vi "CarWashControllerClient.vi"() -> ()   [LabVIEW 2021]
uses:
  CarWashControllerStates.ctl
  <vilib>/regexp/Match Regular Expression.xnode
panel:
  out "error out":errorcluster
  in  "btnStop":bool
  out "tblink 4":bool
  out "tblink 3":bool
  out "tblink 2":bool
  out "tblink1":bool
  out "Seconds":string
  out "Minute":string
  out "Hour":string
  out "AM/PM":string
  out "Date":string
  out "Time":dbl
  out "Remaining Time":dbl
  in  "btnEconomy":bool
  in  "btnDeluxe":bool
  out "carState":string
  in  "LED-VOP":bool
  in  "LED-AD":bool
  in  "LED-CWR":bool
  in  "LED-MHPW":bool
  in  "LED-UBW":bool
  in  "LED-SA":bool
  out "CarWash Details":string
  out "CarWash Bytes":string
  out "Elapsed time":dbl
  in  "Set time":dbl
  in  "Air Dry Position Switch":bool
  in  "Main Wash Position Switch":bool
  in  "Under Body Wash Position \nSwitch":bool
  # "Purchase Selection"
  # "Select Your Wash"
  # "Remaining Time"
  # "Car Wash simulation switch"
  # "Air Dry\nPosition\nSwitch"
  # "Main Wash\nPosition \nSwitch"
  # "Deluxe Wash"
  # "Economy Wash"
  # "Car Wash Indicators"
  # "Under Body Wash"
  # "Soap Application"
  # "Main High Pressure Wash"
  # "Clear Water Rinse"
  # "Air Dry"
  # "Vehicle Out of Position"
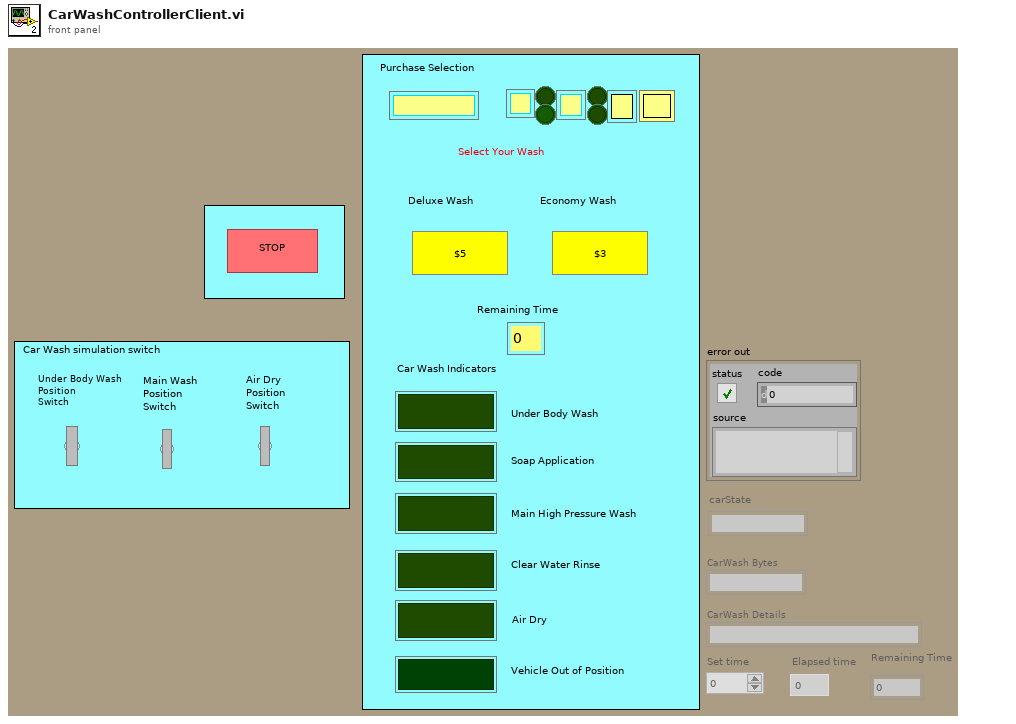
[diagram p1: front panel]
types:
  T1 = typedef "CarWashControllerStates.ctl" = enum16{"Start", "CarWashSelection", "Underbody Wash", "Soap Application", "Main High-Pressure Wash", "Clear Water rinse", "Air Dry Cycle", "Format", "Transmission", "End"}
  T2 = enum8{"Enabled", "Disabled", "Disabled and Grayed Out"}
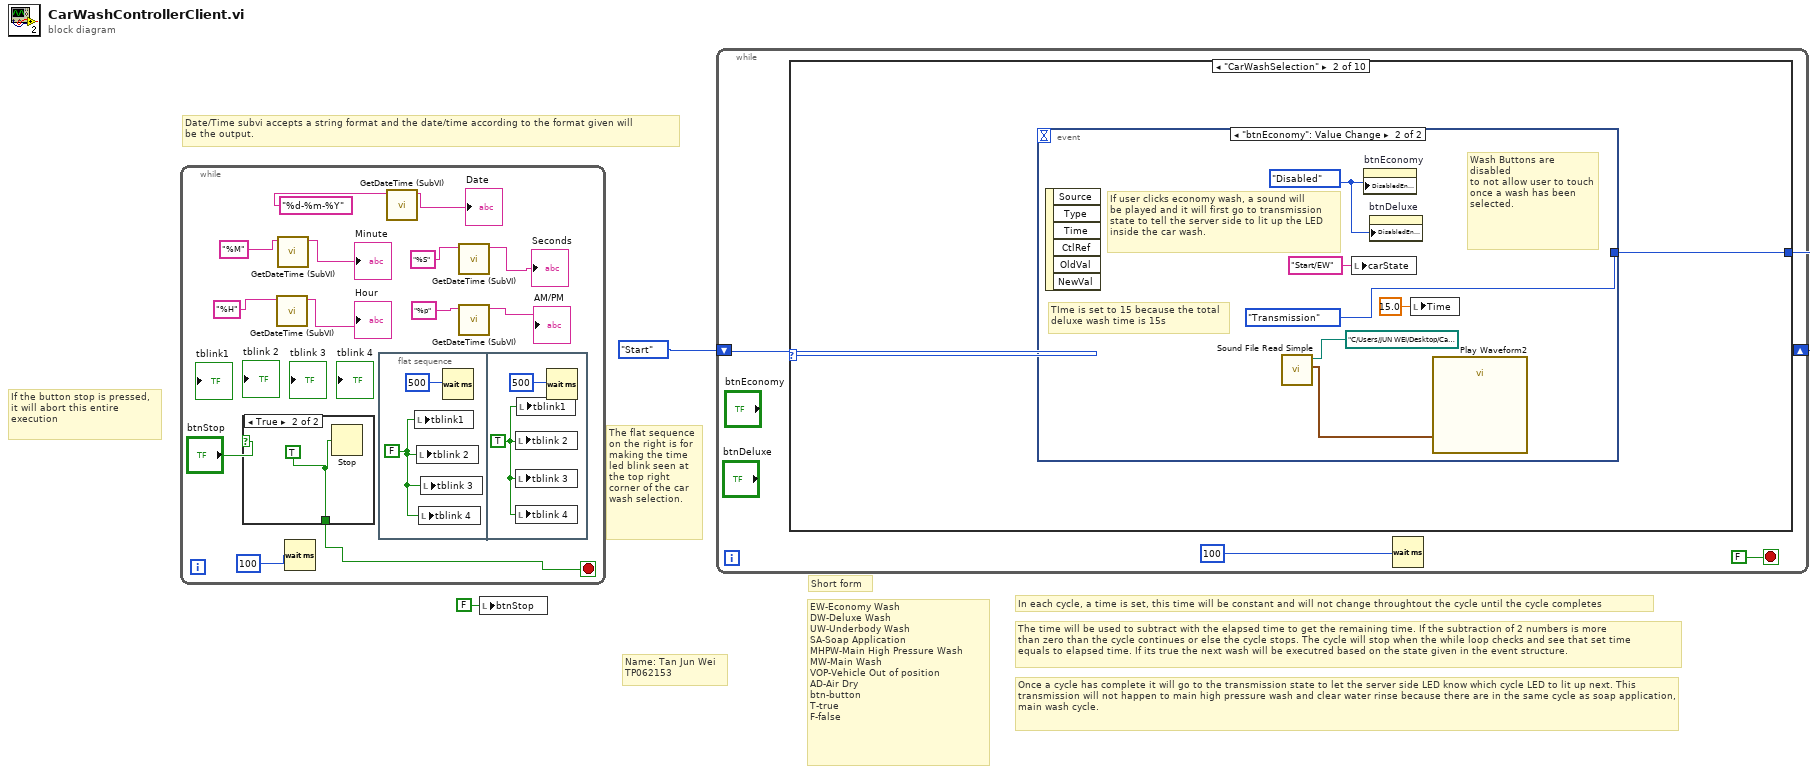
[diagram p0: block diagram]
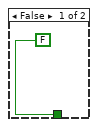
[diagram p2: hidden frame]
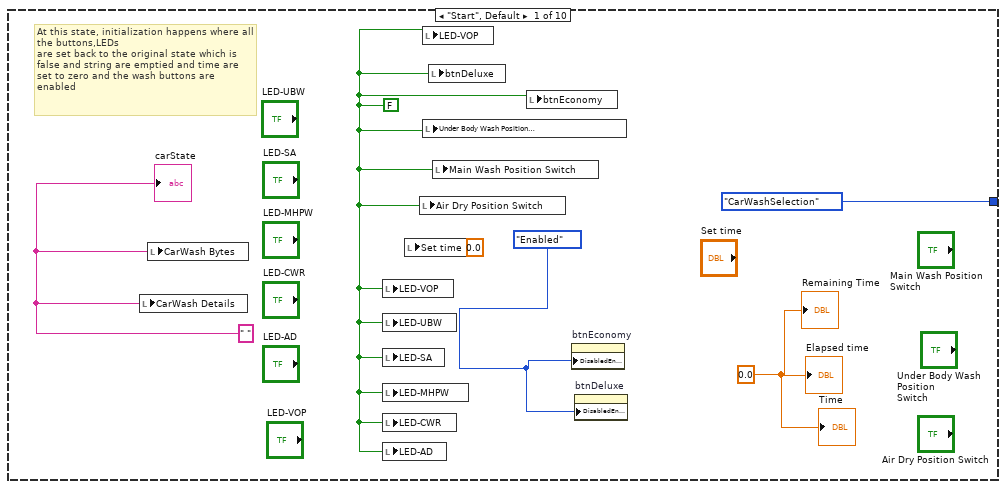
[diagram p3: hidden frame]
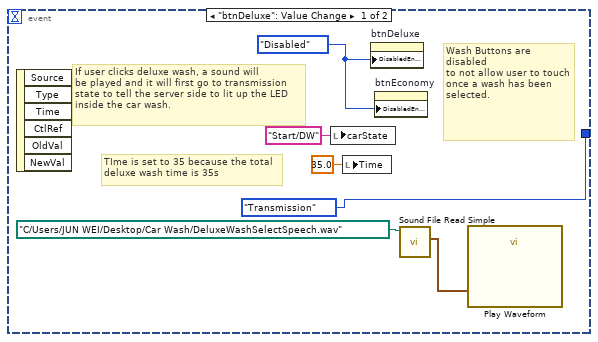
[diagram p4: hidden frame]
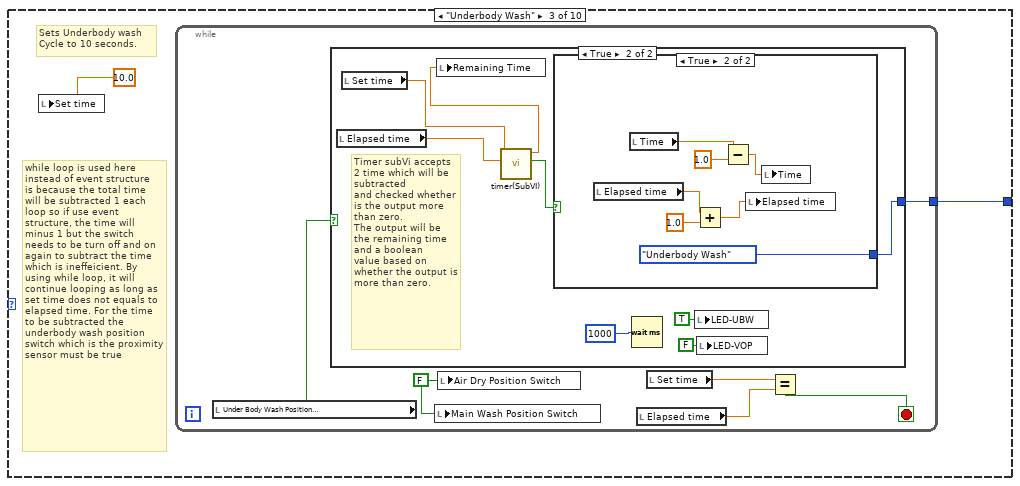
[diagram p5: hidden frame]
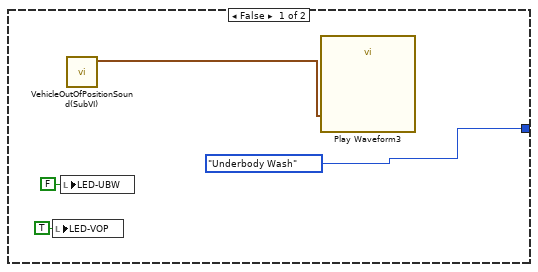
[diagram p6: hidden frame]
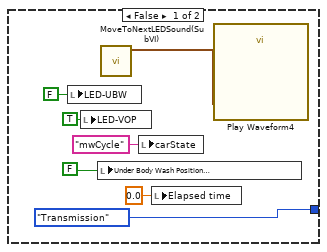
[diagram p7: hidden frame]
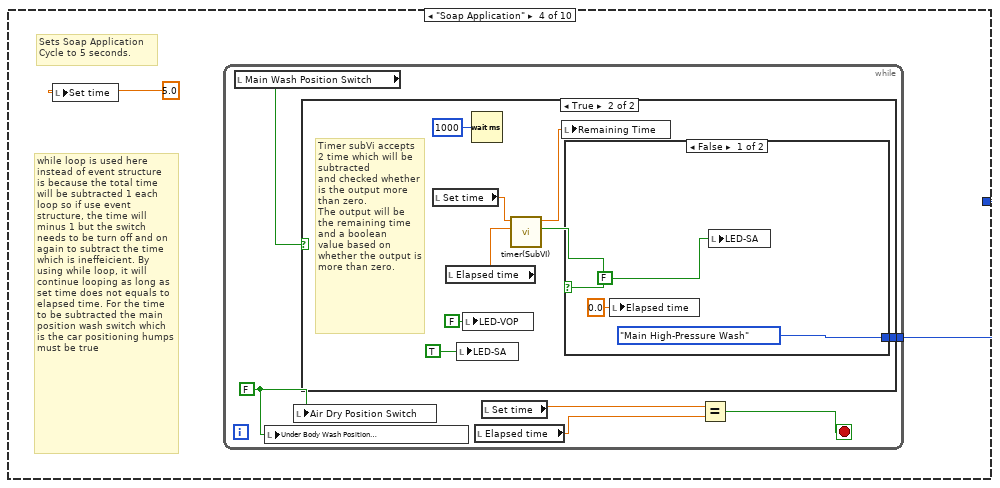
[diagram p8: hidden frame]
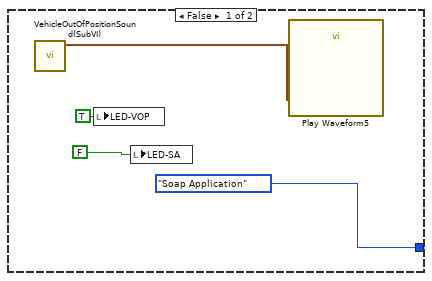
[diagram p9: hidden frame]
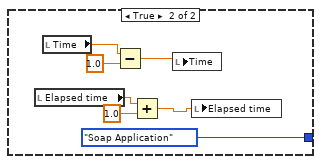
[diagram p10: hidden frame]
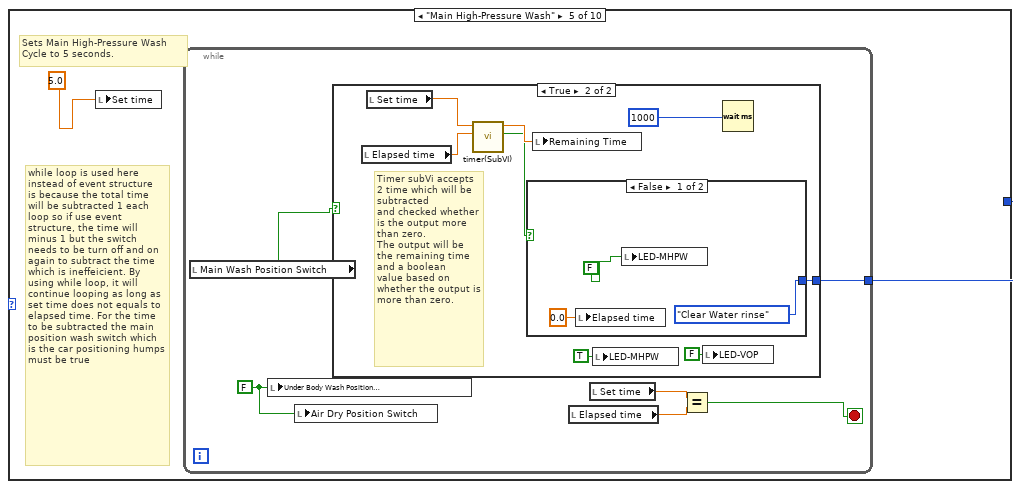
[diagram p11: hidden frame]
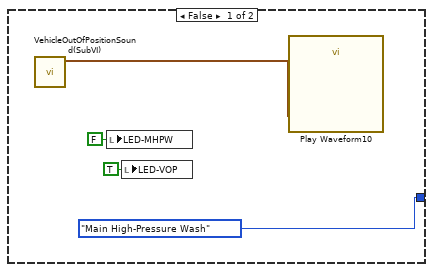
[diagram p12: hidden frame]
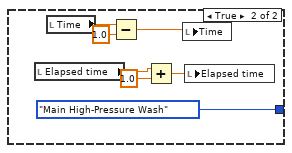
[diagram p13: hidden frame]
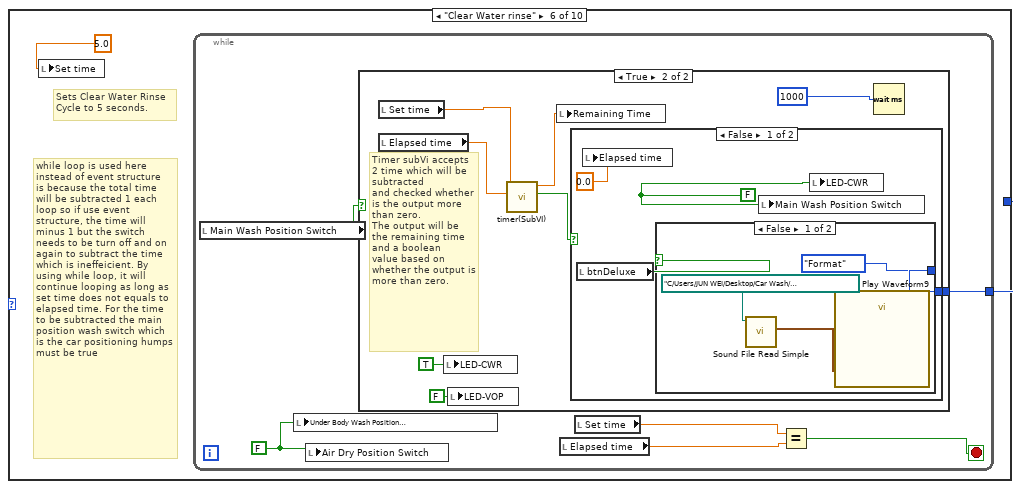
[diagram p14: hidden frame]
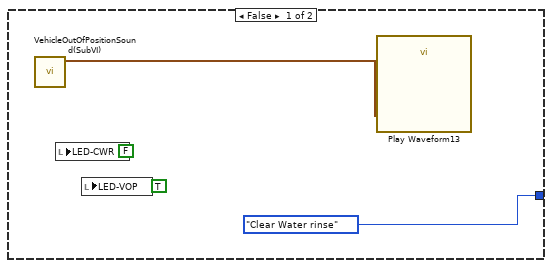
[diagram p15: hidden frame]
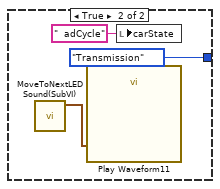
[diagram p16: hidden frame]
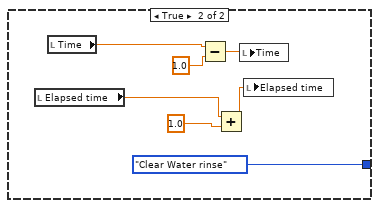
[diagram p17: hidden frame]
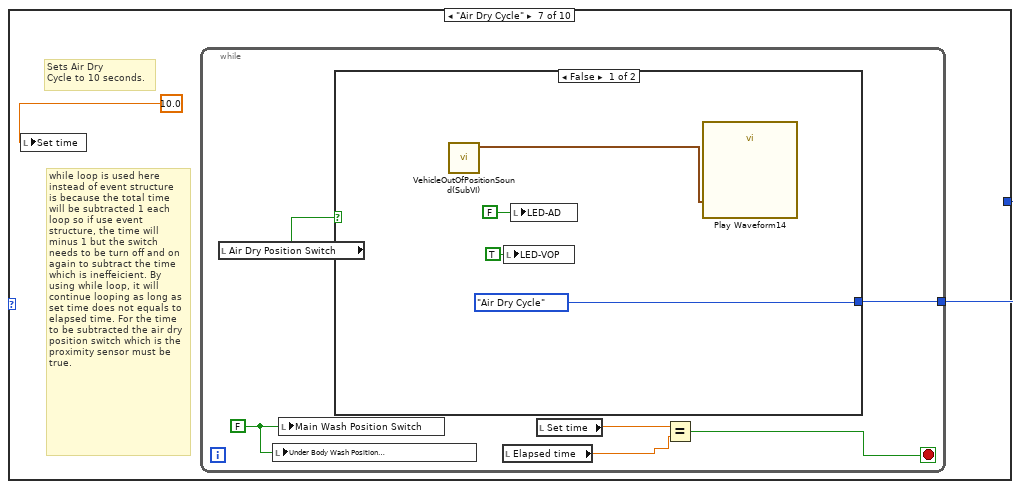
[diagram p18: hidden frame]
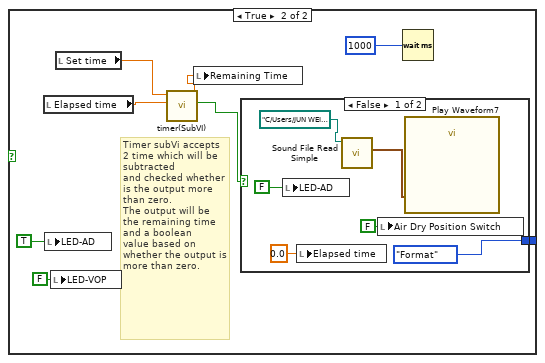
[diagram p19: hidden frame]
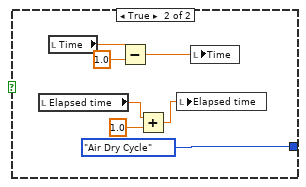
[diagram p20: hidden frame]
diagram:
  # "Short form"
  # "EW-Economy Wash\nDW-Deluxe Wash\nUW-Underbody Wash\nSA-Soap Application\nMHPW-Main High Pressure Wash\nMW-Main Wash\nVOP-Vehicle Out of position\nAD-Air Dry\nbtn-button\nT-true\nF-false"
  # "Name: Tan Jun Wei\nTP062153"
  # "Date/Time subvi accepts a string format and the date/time according to the format given will \nbe the output."
  # "The flat sequence on the right is for making the time led blink seen at the top right corner of the car wash selection."
  # "If the button stop is pressed, it will abort this entire execution"
  # "Once a cycle has complete it will go to the transmission state to let the server side LED know which cycle LED to lit up next. This transmission will not happen to main high pressure wash and clear water rinse because there are in the same cycle as soap application, main wash cycle."
  # "The time will be used to subtract with the elapsed time to get the remaining time. If the subtraction of 2 numbers is more \nthan zero than the cycle continues or else the cycle stops. The cycle will stop when the while loop checks and see that set time\nequals to elapsed time. If its true the next wash will be executred based on the state given in the event structure."
  # "In each cycle, a time is set, this time will be constant and will not change throughtout the cycle until the cycle completes"
  n1 = while {
    stop <- w3 stop-if-true
    n2 = case shown="True" "btnStop" {
      tunnel: [FALSE w17] -> w3
      frame False {
      }
      frame True {
        w17 = TRUE
        n3 = Stop(stop? (T)=w17) -> ()
      }
    }
    n4 = call "GetDateTime (SubVI).vi"("time format string (%c)"="%H") -> ("date/time string"=→"Hour":string)  [unwired: 10 in]
    n5 = call "GetDateTime (SubVI).vi"("time format string (%c)"="%M") -> ("date/time string"=→"Minute":string)  [unwired: 10 in]
    n6 = Wait (ms)(milliseconds to wait=u32 100 ("millisecond timer value")) -> ()  [unwired: 1 out]
    n7 = flat-sequence {
      frame #0 {
        w19 = FALSE ("blink 2")
        n8 = local write "tblink1"(w19) -> ()
        n9 = local write "tblink 2"(w19) -> ()
        n10 = local write "tblink 4"(w19) -> ()
        n11 = local write "tblink 3"(w19) -> ()
        n12 = Wait (ms)(milliseconds to wait=u32 500 ("millisecond timer value")) -> ()  [unwired: 1 out]
      }
      frame #1 {
        w21 = TRUE ("blink 2")
        n13 = local write "tblink 2"(w21) -> ()
        n14 = local write "tblink 3"(w21) -> ()
        n15 = local write "tblink 4"(w21) -> ()
        n16 = local write "tblink1"(w21) -> ()
        n17 = Wait (ms)(milliseconds to wait=u32 500 ("millisecond timer value")) -> ()  [unwired: 1 out]
      }
    }
    n18 = call "GetDateTime (SubVI).vi"("time format string (%c)"="%d-%m-%Y") -> ("date/time string"=→"Date":string)  [unwired: 10 in]
    n19 = call "GetDateTime (SubVI).vi"("time format string (%c)"="%S") -> ("date/time string"=→"Seconds":string)  [unwired: 10 in]
    n20 = call "GetDateTime (SubVI).vi"("time format string (%c)"="%p") -> ("date/time string"=→"AM/PM":string)  [unwired: 10 in]
  }
  n21 = local write "btnStop"(FALSE ("btnStop")) -> ()
  n22 = while {
    shift-right: [w23] -> _
    shift-left: CarWashControllerStates."Start" -> [w25]
    stop <- FALSE stop-if-true
    n23 = case shown="\"CarWashSelection\"" w25 {
      tunnel: [CarWashControllerStates."CarWashSelection" w32 w46 w79 w109 w139 w176 CarWashControllerStates."Transmission" w230 CarWashControllerStates."Start"] -> w23
      frame "Start", Default {
        w27 = 0.0 ("Remaining Time")
        w28 = " " ("carState")
        w29 = T2."Enabled" ("Disabled")
        w26 = FALSE ("btnEconomy")
        # "At this state, initialization happens where all the buttons,LEDs\nare set back to the original state which is false and string are emptied and time are set to zero and the wash buttons are enabled"
        n24 = local write "CarWash Details"(w28) -> ()
        n25 = local write "CarWash Bytes"(w28) -> ()
        n26 = local write "LED-VOP"(w26) -> ()
        n27 = local write "LED-UBW"(w26) -> ()
        n28 = local write "LED-SA"(w26) -> ()
        n29 = local write "LED-MHPW"(w26) -> ()
        n30 = local write "LED-CWR"(w26) -> ()
        n31 = local write "LED-AD"(w26) -> ()
        n32 = local write "Set time"(0.0 ("Set time")) -> ()
        n33 = local write "Air Dry Position Switch"(w26) -> ()
        n34 = local write "LED-VOP"(w26) -> ()
        n35 = local write "Under Body Wash Position \nSwitch"(w26) -> ()
        n36 = local write "btnDeluxe"(w26) -> ()
        n37 = local write "Main Wash Position Switch"(w26) -> ()
        n38 = local write "btnEconomy"(w26) -> ()
        n39 = property on="btnEconomy" class="Bool (strict)"("DisabledEnum"=w29) -> ()  [unwired: 2 in, 2 out]
        n40 = property on="btnDeluxe" class="Bool (strict)"("DisabledEnum"=w29) -> ()  [unwired: 2 in, 2 out]
        "carState" <- w28
        "Remaining Time" <- w27
        "Elapsed time" <- w27
        "Time" <- w27
      }
      frame "CarWashSelection" {
        n41 = event shown="[1] \"btnEconomy\": Value Change" {
          selector: _ -> [_ _]
          dyn-events: _ -> [_ _]
          timeout: _ -> [_ _]
          tunnel: [CarWashControllerStates."Transmission" CarWashControllerStates."Transmission"] -> w32
          event "btnDeluxe": Value Change {
            w35 = T2."Disabled" ("Disabled")
            # "TIme is set to 35 because the total\ndeluxe wash time is 35s"
            # "Wash Buttons are disabled\nto not allow user to touch once a wash has been selected."
            # "If user clicks deluxe wash, a sound will\nbe played and it will first go to transmission\nstate to tell the server side to lit up the LED \ninside the car wash."
            n42 = event-data() -> ()  [unwired: 1 in, 6 out]
            n43 = local write "carState"("Start/DW" ("carState")) -> ()
            n44 = local write "Time"(35.0 ("Time")) -> ()
            n45 = property on="btnDeluxe" class="Bool (strict)"("DisabledEnum"=w35) -> ()  [unwired: 2 in, 2 out]
            n46 = property on="btnEconomy" class="Bool (strict)"("DisabledEnum"=w35) -> ()  [unwired: 2 in, 2 out]
            n47 = call <vilib>:"Sound File Read Simple.vi"("path"=path "C:/Users/JUN WEI/Desktop/Car Wash/DeluxeWashSelectSpeech.wav") -> ("data"=w33:waveform(dbl)[])  [unwired: 7 in, 3 out]
            n48 = call "Play Waveform"("Data"=w33) -> ()  [unwired: 18 in, 1 out]
          }
          event "btnEconomy": Value Change {
            w41 = T2."Disabled" ("Disabled")
            # "TIme is set to 15 because the total\ndeluxe wash time is 15s"
            # "Wash Buttons are disabled\nto not allow user to touch once a wash has been selected."
            # "If user clicks economy wash, a sound will\nbe played and it will first go to transmission\nstate to tell the server side to lit up the LED \ninside the car wash."
            n49 = event-data() -> ()  [unwired: 1 in, 6 out]
            n50 = call <vilib>:"Sound File Read Simple.vi"("path"=path "C:/Users/JUN WEI/Desktop/Car Wash/EconomyWashSelectSpeech.wav") -> ("data"=w40:waveform(dbl)[])  [unwired: 7 in, 3 out]
            n51 = local write "carState"("Start/EW" ("carState")) -> ()
            n52 = property on="btnEconomy" class="Bool (strict)"("DisabledEnum"=w41) -> ()  [unwired: 2 in, 2 out]
            n53 = property on="btnDeluxe" class="Bool (strict)"("DisabledEnum"=w41) -> ()  [unwired: 2 in, 2 out]
            n54 = local write "Time"(15.0 ("Time")) -> ()
            n55 = call "Play Waveform2"("Data"=w40) -> ()  [unwired: 18 in, 1 out]
          }
        }
      }
      frame "Underbody Wash" {
        # "Sets Underbody wash \nCycle to 10 seconds."
        # "while loop is used here\ninstead of event structure\nis because the total time will be subtracted 1 each loop so if use event structure, the time will  minus 1 but the switch needs to be turn off and on again to subtract the time which is ineffeicient. By using while loop, it will continue looping as long as set time does not equals to elapsed time. For the time to be subtracted the underbody wash position switch which is the proximity sensor must be true"
        n56 = local write "Set time"(10.0 ("Set time")) -> ()
        n57 = while {
          tunnel: [w51] -> w46
          stop <- w48 stop-if-true
          w47 = FALSE ("Air Dry Position Switch")
          n58 = local read "Under Body Wash Position \nSwitch"() -> (w52:bool)
          n59 = case shown="True" w52 {
            tunnel: [CarWashControllerStates."Underbody Wash" w57] -> w51
            frame False {
              n60 = local write "LED-VOP"(TRUE ("swVOP")) -> ()
              n61 = local write "LED-UBW"(FALSE ("Boolean")) -> ()
              n62 = call "VehicleOutOfPositionSound(SubVI).vi"() -> ("data"=w53:waveform(dbl)[])  [unwired: 11 in]
              n63 = call "Play Waveform3"("Data"=w53) -> ()  [unwired: 18 in, 1 out]
            }
            frame True {
              # "Timer subVi accepts\n2 time which will be subtracted\nand checked whether is the output more than zero.\nThe output will be the remaining time and a boolean \nvalue based on whether the output is more than zero."
              n64 = local read "Elapsed time"() -> (w63:dbl)
              n65 = local read "Set time"() -> (w64:dbl)
              n66 = call "timer(SubVI).vi"("Elapsed time"=w63, "Set time"=w64) -> ("Boolean"=w61:bool, "Remaining Time"=w62:dbl)  [unwired: 8 in]
              n67 = local write "Remaining Time"(w62) -> ()
              n68 = case shown="True" w61 {
                tunnel: [CarWashControllerStates."Transmission" CarWashControllerStates."Underbody Wash"] -> w57
                frame False {
                  n69 = local write "LED-UBW"(FALSE ("LED-UBW")) -> ()
                  n70 = local write "LED-VOP"(TRUE ("swVOP")) -> ()
                  n71 = local write "Under Body Wash Position \nSwitch"(FALSE ("s1")) -> ()
                  n72 = call "MoveToNextLEDSound(SubVI).vi"() -> ("data"=w65:waveform(dbl)[])  [unwired: 11 in]
                  n73 = local write "carState"("mwCycle" ("carState")) -> ()
                  n74 = local write "Elapsed time"(0.0 ("Elapsed time")) -> ()
                  n75 = call "Play Waveform4"("Data"=w65) -> ()  [unwired: 18 in, 1 out]
                }
                frame True {
                  n76 = local read "Elapsed time"() -> (w77:dbl)
                  n77 = local read "Time"() -> (w73:dbl)
                  n78 = Add(x=w77, y=1.0) -> (x+y=w76:dbl)
                  n79 = Subtract(x=w73, y=1.0) -> (x-y=w74:dbl)
                  n80 = local write "Elapsed time"(w76) -> ()
                  n81 = local write "Time"(w74) -> ()
                }
              }
              n82 = Wait (ms)(milliseconds to wait=u32 1000 ("millisecond timer value")) -> ()  [unwired: 1 out]
              n83 = local write "LED-UBW"(TRUE ("Boolean")) -> ()
              n84 = local write "LED-VOP"(FALSE ("swVOP")) -> ()
            }
          }
          n85 = local write "Main Wash Position Switch"(w47) -> ()
          n86 = local write "Air Dry Position Switch"(w47) -> ()
          n87 = local read "Elapsed time"() -> (w49:dbl)
          n88 = local read "Set time"() -> (w50:dbl)
          n89 = Equal?(x=w50, y=w49) -> (x = y?=w48:bool)
        }
      }
      frame "Soap Application" {
        # "Sets Soap Application \nCycle to 5 seconds."
        # "while loop is used here\ninstead of event structure\nis because the total time will be subtracted 1 each loop so if use event structure, the time will  minus 1 but the switch needs to be turn off and on again to subtract the time which is ineffeicient. By using while loop, it will continue looping as long as set time does not equals to elapsed time. For the time to be subtracted the main position wash switch which is the car positioning humps must be true"
        n90 = local write "Set time"(5.0 ("Set time")) -> ()
        n91 = while {
          tunnel: [w85] -> w79
          stop <- w82 stop-if-true
          w81 = FALSE ("Air Dry Position Switch")
          n92 = local read "Main Wash Position Switch"() -> (w86:bool)
          n93 = local write "Under Body Wash Position \nSwitch"(w81) -> ()
          n94 = local write "Air Dry Position Switch"(w81) -> ()
          n95 = case shown="True" w86 {
            tunnel: [CarWashControllerStates."Soap Application" w98] -> w85
            frame False {
              n96 = call "VehicleOutOfPositionSound(SubVI).vi"() -> ("data"=w87:waveform(dbl)[])  [unwired: 11 in]
              n97 = local write "LED-VOP"(TRUE ("swVOP")) -> ()
              n98 = local write "LED-SA"(FALSE ("Boolean")) -> ()
              n99 = call "Play Waveform5"("Data"=w87) -> ()  [unwired: 18 in, 1 out]
            }
            frame True {
              # "Timer subVi accepts\n2 time which will be subtracted\nand checked whether is the output more than zero.\nThe output will be the remaining time and a boolean \nvalue based on whether the output is more than zero."
              n100 = local read "Set time"() -> (w93:dbl)
              n101 = local read "Elapsed time"() -> (w94:dbl)
              n102 = local write "LED-SA"(TRUE ("Boolean 2")) -> ()
              n103 = local write "LED-VOP"(FALSE ("swVOP")) -> ()
              n104 = Wait (ms)(milliseconds to wait=u32 1000) -> ()  [unwired: 1 out]
              n105 = call "timer(SubVI).vi"("Elapsed time"=w94, "Set time"=w93) -> ("Boolean"=w91:bool, "Remaining Time"=w92:dbl)  [unwired: 8 in]
              n106 = local write "Remaining Time"(w92) -> ()
              n107 = case shown="False" w91 {
                tunnel: [CarWashControllerStates."Main High-Pressure Wash" CarWashControllerStates."Soap Application"] -> w98
                frame False {
                  n108 = local write "Elapsed time"(0.0 ("Elapsed time")) -> ()
                  n109 = local write "LED-SA"(FALSE ("s2")) -> ()
                }
                frame True {
                  n110 = local read "Elapsed time"() -> (w108:dbl)
                  n111 = local read "Time"() -> (w104:dbl)
                  n112 = Subtract(x=w104, y=1.0) -> (x-y=w102:dbl)
                  n113 = Add(x=w108, y=1.0) -> (x+y=w106:dbl)
                  n114 = local write "Time"(w102) -> ()
                  n115 = local write "Elapsed time"(w106) -> ()
                }
              }
            }
          }
          n116 = local read "Elapsed time"() -> (w83:dbl)
          n117 = local read "Set time"() -> (w84:dbl)
          n118 = Equal?(x=w84, y=w83) -> (x = y?=w82:bool)
        }
      }
      frame "Main High-Pressure Wash" {
        # "Sets Main High-Pressure Wash \nCycle to 5 seconds."
        # "while loop is used here\ninstead of event structure\nis because the total time will be subtracted 1 each loop so if use event structure, the time will  minus 1 but the switch needs to be turn off and on again to subtract the time which is ineffeicient. By using while loop, it will continue looping as long as set time does not equals to elapsed time. For the time to be subtracted the main position wash switch which is the car positioning humps must be true"
        n119 = local write "Set time"(5.0 ("Set time")) -> ()
        n120 = while {
          tunnel: [w113] -> w109
          stop <- w114 stop-if-true
          w111 = FALSE ("Under Body Wash Position \nSwitch")
          n121 = local read "Main Wash Position Switch"() -> (w112:bool)
          n122 = local write "Under Body Wash Position \nSwitch"(w111) -> ()
          n123 = local write "Air Dry Position Switch"(w111) -> ()
          n124 = case shown="True" w112 {
            tunnel: [CarWashControllerStates."Main High-Pressure Wash" w127] -> w113
            frame False {
              n125 = call "VehicleOutOfPositionSound(SubVI).vi"() -> ("data"=w117:waveform(dbl)[])  [unwired: 11 in]
              n126 = local write "LED-MHPW"(FALSE ("Boolean 3")) -> ()
              n127 = local write "LED-VOP"(TRUE ("swVOP")) -> ()
              n128 = call "Play Waveform10"("Data"=w117) -> ()  [unwired: 18 in, 1 out]
            }
            frame True {
              # "Timer subVi accepts\n2 time which will be subtracted\nand checked whether is the output more than zero.\nThe output will be the remaining time and a boolean \nvalue based on whether the output is more than zero."
              n129 = local read "Elapsed time"() -> (w124:dbl)
              n130 = local read "Set time"() -> (w123:dbl)
              n131 = call "timer(SubVI).vi"("Elapsed time"=w124, "Set time"=w123) -> ("Boolean"=w121:bool, "Remaining Time"=w122:dbl)  [unwired: 8 in]
              n132 = case shown="False" w121 {
                tunnel: [CarWashControllerStates."Clear Water rinse" CarWashControllerStates."Main High-Pressure Wash"] -> w127
                frame False {
                  n133 = local write "Elapsed time"(0.0 ("Elapsed time")) -> ()
                  n134 = local write "LED-MHPW"(FALSE ("s2")) -> ()
                }
                frame True {
                  n135 = local read "Elapsed time"() -> (w137:dbl)
                  n136 = local read "Time"() -> (w135:dbl)
                  n137 = Subtract(x=w135, y=1.0) -> (x-y=w132:dbl)
                  n138 = Add(x=w137, y=1.0) -> (x+y=w133:dbl)
                  n139 = local write "Time"(w132) -> ()
                  n140 = local write "Elapsed time"(w133) -> ()
                }
              }
              n141 = local write "Remaining Time"(w122) -> ()
              n142 = local write "LED-MHPW"(TRUE ("Boolean 3")) -> ()
              n143 = local write "LED-VOP"(FALSE ("swVOP")) -> ()
              n144 = Wait (ms)(milliseconds to wait=u32 1000 ("millisecond timer value")) -> ()  [unwired: 1 out]
            }
          }
          n145 = local read "Elapsed time"() -> (w115:dbl)
          n146 = local read "Set time"() -> (w116:dbl)
          n147 = Equal?(x=w116, y=w115) -> (x = y?=w114:bool)
        }
      }
      frame "Clear Water rinse" {
        # "while loop is used here\ninstead of event structure\nis because the total time will be subtracted 1 each loop so if use event structure, the time will  minus 1 but the switch needs to be turn off and on again to subtract the time which is ineffeicient. By using while loop, it will continue looping as long as set time does not equals to elapsed time. For the time to be subtracted the main position wash switch which is the car positioning humps must be true"
        # "Sets Clear Water Rinse \nCycle to 5 seconds."
        n148 = local write "Set time"(5.0 ("Set time")) -> ()
        n149 = while {
          tunnel: [w142] -> w139
          stop <- w144 stop-if-true
          w141 = FALSE ("Air Dry Position Switch")
          n150 = local read "Main Wash Position Switch"() -> (w143:bool)
          n151 = local write "Under Body Wash Position \nSwitch"(w141) -> ()
          n152 = local write "Air Dry Position Switch"(w141) -> ()
          n153 = case shown="True" w143 {
            tunnel: [CarWashControllerStates."Clear Water rinse" w156] -> w142
            frame False {
              n154 = call "VehicleOutOfPositionSound(SubVI).vi"() -> ("data"=w147:waveform(dbl)[])  [unwired: 11 in]
              n155 = local write "LED-CWR"(FALSE ("Boolean 4")) -> ()
              n156 = local write "LED-VOP"(TRUE ("swVOP")) -> ()
              n157 = call "Play Waveform13"("Data"=w147) -> ()  [unwired: 18 in, 1 out]
            }
            frame True {
              # "Timer subVi accepts\n2 time which will be subtracted\nand checked whether is the output more than zero.\nThe output will be the remaining time and a boolean \nvalue based on whether the output is more than zero."
              n158 = local read "Set time"() -> (w151:dbl)
              n159 = local read "Elapsed time"() -> (w152:dbl)
              n160 = local write "LED-CWR"(TRUE ("Boolean 4")) -> ()
              n161 = local write "LED-VOP"(FALSE ("swVOP")) -> ()
              n162 = call "timer(SubVI).vi"("Elapsed time"=w152, "Set time"=w151) -> ("Boolean"=w154:bool, "Remaining Time"=w153:dbl)  [unwired: 8 in]
              n163 = local write "Remaining Time"(w153) -> ()
              n164 = case shown="False" w154 {
                tunnel: [w162 CarWashControllerStates."Clear Water rinse"] -> w156
                frame False {
                  w161 = FALSE ("s2")
                  n165 = local read "btnDeluxe"() -> (w160:bool)
                  n166 = local write "Elapsed time"(0.0 ("Elapsed time")) -> ()
                  n167 = case shown="False" w160 {
                    tunnel: [CarWashControllerStates."Format" CarWashControllerStates."Transmission"] -> w162
                    frame False {
                      n168 = call <vilib>:"Sound File Read Simple.vi"("path"=path "C:/Users/JUN WEI/Desktop/Car Wash/EconomyWashExitSpeech.wav") -> ("data"=w164:waveform(dbl)[])  [unwired: 7 in, 3 out]
                      n169 = call "Play Waveform9"("Data"=w164) -> ()  [unwired: 18 in, 1 out]
                    }
                    frame True {
                      n170 = call "MoveToNextLEDSound(SubVI).vi"() -> ("data"=w166:waveform(dbl)[])  [unwired: 11 in]
                      n171 = call "Play Waveform11"("Data"=w166) -> ()  [unwired: 18 in, 1 out]
                      n172 = local write "carState"("  adCycle" ("carState")) -> ()
                    }
                  }
                  n173 = local write "Main Wash Position Switch"(w161) -> ()
                  n174 = local write "LED-CWR"(w161) -> ()
                }
                frame True {
                  n175 = local read "Elapsed time"() -> (w174:dbl)
                  n176 = local read "Time"() -> (w170:dbl)
                  n177 = Subtract(x=w170, y=1.0) -> (x-y=w171:dbl)
                  n178 = Add(x=w174, y=1.0) -> (x+y=w173:dbl)
                  n179 = local write "Time"(w171) -> ()
                  n180 = local write "Elapsed time"(w173) -> ()
                }
              }
              n181 = Wait (ms)(milliseconds to wait=u32 1000 ("millisecond timer value")) -> ()  [unwired: 1 out]
            }
          }
          n182 = local read "Elapsed time"() -> (w145:dbl)
          n183 = local read "Set time"() -> (w146:dbl)
          n184 = Equal?(x=w146, y=w145) -> (x = y?=w144:bool)
        }
      }
      frame "Air Dry Cycle" {
        # "Sets Air Dry  \nCycle to 10 seconds."
        # "while loop is used here\ninstead of event structure\nis because the total time will be subtracted 1 each loop so if use event structure, the time will  minus 1 but the switch needs to be turn off and on again to subtract the time which is ineffeicient. By using while loop, it will continue looping as long as set time does not equals to elapsed time. For the time to be subtracted the air dry position switch which is the proximity sensor must be true."
        n185 = local write "Set time"(10.0 ("Set time")) -> ()
        n186 = while {
          tunnel: [w182] -> w176
          stop <- w179 stop-if-true
          w178 = FALSE ("Main Wash Position Switch")
          n187 = local read "Air Dry Position Switch"() -> (w183:bool)
          n188 = local write "Under Body Wash Position \nSwitch"(w178) -> ()
          n189 = local write "Main Wash Position Switch"(w178) -> ()
          n190 = case shown="False" w183 {
            tunnel: [CarWashControllerStates."Air Dry Cycle" w194] -> w182
            frame False {
              n191 = call "VehicleOutOfPositionSound(SubVI).vi"() -> ("data"=w184:waveform(dbl)[])  [unwired: 11 in]
              n192 = local write "LED-VOP"(TRUE ("swVOP")) -> ()
              n193 = local write "LED-AD"(FALSE ("Boolean 5")) -> ()
              n194 = call "Play Waveform14"("Data"=w184) -> ()  [unwired: 18 in, 1 out]
            }
            frame True {
              # "Timer subVi accepts\n2 time which will be subtracted\nand checked whether is the output more than zero.\nThe output will be the remaining time and a boolean \nvalue based on whether the output is more than zero."
              n195 = local read "Elapsed time"() -> (w189:dbl)
              n196 = local write "LED-AD"(TRUE ("Boolean 5")) -> ()
              n197 = local write "LED-VOP"(FALSE ("swVOP")) -> ()
              n198 = local read "Set time"() -> (w188:dbl)
              n199 = call "timer(SubVI).vi"("Elapsed time"=w189, "Set time"=w188) -> ("Boolean"=w191:bool, "Remaining Time"=w190:dbl)  [unwired: 8 in]
              n200 = local write "Remaining Time"(w190) -> ()
              n201 = case shown="False" w191 {
                tunnel: [CarWashControllerStates."Format" CarWashControllerStates."Air Dry Cycle"] -> w194
                frame False {
                  n202 = local write "LED-AD"(FALSE ("Boolean 5")) -> ()
                  n203 = local write "Elapsed time"(0.0 ("Elapsed time")) -> ()
                  n204 = call <vilib>:"Sound File Read Simple.vi"("path"=path "C:/Users/JUN WEI/Desktop/Car Wash/DeluxeWashExitSpeech.wav") -> ("data"=w196:waveform(dbl)[])  [unwired: 7 in, 3 out]
                  n205 = local write "Air Dry Position Switch"(FALSE ("s3")) -> ()
                  n206 = call "Play Waveform7"("Data"=w196) -> ()  [unwired: 18 in, 1 out]
                }
                frame True {
                  n207 = local read "Elapsed time"() -> (w208:dbl)
                  n208 = local read "Time"() -> (w203:dbl)
                  n209 = Subtract(x=w203, y=1.0) -> (x-y=w202:dbl)
                  n210 = Add(x=w208, y=1.0) -> (x+y=w206:dbl)
                  n211 = local write "Elapsed time"(w206) -> ()
                  n212 = local write "Time"(w202) -> ()
                }
              }
              n213 = Wait (ms)(milliseconds to wait=u32 1000 ("millisecond timer value")) -> ()  [unwired: 1 out]
            }
          }
          n214 = local read "Elapsed time"() -> (w180:dbl)
          n215 = local read "Set time"() -> (w181:dbl)
          n216 = Equal?(x=w181, y=w180) -> (x = y?=w179:bool)
        }
      }
      frame "Format" {
        w210 = "End" ("carState")
        # "The car state is set to End and concatenated to the car wash details is because this is to tell the server side LED that the car wash is over and is ready for the next customer."
        # "This is to which button\nwas pressed and based on it, the type of wash will be set accordingly.\nIn this case if button economy is pressed the case structure will be true so the string Economy wash will be concatenated."
        # "At this stage the car wash details is formatted according to the requirements where its date time and type of wash."
        n217 = local read "btnEconomy"() -> (w225:bool)
        n218 = Get Date/Time In Seconds() -> (seconds since 1Jan1904=w223:timestamp)
        n219 = case shown="False" w225 {
          tunnel: ["Deluxe Wash" "Economy Wash" ("string")] -> w212
          frame False {
          }
          frame True {
          }
        }
        n220 = Get Date/Time In Seconds() -> (seconds since 1Jan1904=w224:timestamp)
        n221 = Format Date/Time String(time format string (%c)="%H:%M:%S", seconds (now)=w223) -> (date/time string=w221:string)  [unwired: 1 in]
        n222 = Format Date/Time String(time format string (%c)="%d/%m/%Y", seconds (now)=w224) -> (date/time string=w222:string)  [unwired: 1 in]
        n223 = Concatenate Strings(w210, "/" ("string"), w222, "," ("string"), w221, "," ("string"), w212) -> (w218:string)
        "CarWash Details" <- w218
        n224 = local write "carState"(w210) -> ()
        n225 = String Length(string=w218) -> (length=w220:i32)
        n226 = Number To Decimal String(number=w220, width (-)=i16 3) -> (decimal integer string=→"CarWash Bytes":string)
      }
      frame "Transmission" {
        # "The case structure on the right is used to check if the total \ncar wash time(Time) is equals to 0. If equals to zero then it will go to the false case\nand the end state will be executed which means the car wash has been completed.\nIf Time is not equals to 0 then the carState string will be checked with the case structure\nto start the cycle."
        # "The case structure on the left is used to transmit the current cycle the\ncar is in."
        n227 = local read "carState"() -> (w234:string)
        n228 = TCP Open Connection(remote port or service name=u16 7777, timeout ms (60000)=60000) -> (connection ID=w243:refnum<k5>, error out=w240:errorcluster)  [unwired: 3 in]
        n229 = xnode ("Match Regular Expression")("input string"=w234, "regular expression"="/") -> ("before match"=w229:string, "after match"=w232:string)  [unwired: 4 in, 3 out]
        n230 = case shown="\"Start\"" w229 {
          selector: w229 -> [_ _ w503 w507]
          tunnel: [w494 w498 w504 w508] -> w237
          tunnel: [w493 w495 " mwCycle" ("after match") w507] -> w236
          tunnel: w232 -> [_ w496 _ _]
          frame "End", Default {
            n231 = local read "CarWash Bytes"() -> (w494:string)
            n232 = local read "CarWash Details"() -> (w493:string)
          }
          frame "Start" {
            n233 = Concatenate Strings(" Start" ("string"), "/" ("string"), w496) -> (w495:string)
            n234 = String Length(string=w495) -> (length=w499:i32)
            n235 = Number To Decimal String(number=w499, width (-)=i16 2) -> (decimal integer string=w498:string)
          }
          frame "mwCycle" {
            n236 = String Length(string=w503) -> (length=w506:i32)
            n237 = Number To Decimal String(number=w506, width (-)=i16 2) -> (decimal integer string=w504:string)
          }
          frame "  adCycle" {
            n238 = String Length(string=w507) -> (length=w509:i32)
            n239 = Number To Decimal String(number=w509) -> (decimal integer string=w508:string)  [unwired: 1 in]
          }
        }
        n240 = TCP Write(connection ID=w243, data in=w237, error in (no error)=w240) -> (connection ID out=w242:refnum<k5>, error out=w239:errorcluster)  [unwired: 1 in, 1 out]
        n241 = TCP Write(connection ID=w242, data in=w236, error in (no error)=w239) -> (connection ID out=w241:refnum<k5>, error out=w238:errorcluster)  [unwired: 1 in, 1 out]
        n242 = local read "Time"() -> (w235:dbl)
        n243 = TCP Close Connection(connection ID=w241, error in (no error)=w238) -> (error out=→"error out":errorcluster)  [unwired: 1 in, 1 out]
        n244 = Equal To 0?(x=w235) -> (x = 0?=w231:bool)
        n245 = case shown="True" w231 {
          tunnel: [w364 CarWashControllerStates."End"] -> w230
          frame False {
            n246 = local read "carState"() -> (w366:string)
            n247 = xnode "Match Regular Expression"("input string"=w366, "regular expression"="/") -> ("before match"=w367:string, "after match"=w365:string)  [unwired: 4 in, 3 out]
            n248 = case shown="\"mwCycle\"" w367 {
              tunnel: w365 -> [_ _ _ w489]
              tunnel: [CarWashControllerStates."Soap Application" CarWashControllerStates."End" CarWashControllerStates."Air Dry Cycle" w488] -> w364
              frame "mwCycle" {
              }
              frame "End" {
              }
              frame "  adCycle" {
              }
              frame "Start", Default {
                n249 = case shown="\"EW\", Default" w489 {
                  tunnel: [CarWashControllerStates."Soap Application" CarWashControllerStates."Underbody Wash"] -> w488
                  frame "EW", Default {
                  }
                  frame "DW" {
                  }
                }
              }
            }
          }
          frame True {
          }
        }
      }
      frame "End" {
      }
    }
    n250 = Wait (ms)(milliseconds to wait=u32 100 ("millisecond timer value")) -> ()  [unwired: 1 out]
  }
